vi "Get TableName.vi"(8 "error in (no error)":errorcluster caption="entrée d'erreur (pas d'erreur)", 11 "Database Drivers en entrée":refnum<class "Database Drivers.lvclass">) -> (0 "error out":errorcluster caption="sortie d'erreur", 2 "TableName":string, 3 "Database Drivers en sortie":refnum<class "Database Drivers.lvclass">)   [LabVIEW 2020, in "Library Instrument & Equipement.lvlib" / "Library Database.lvlib" / "Database Drivers.lvclass"]
uses:
  Database Drivers.lvclass
  Database Drivers.lvclass/Database Drivers.ctl
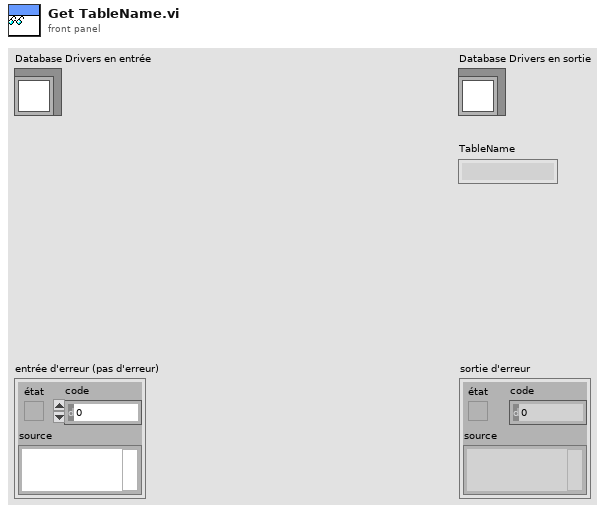
[diagram p1: front panel]
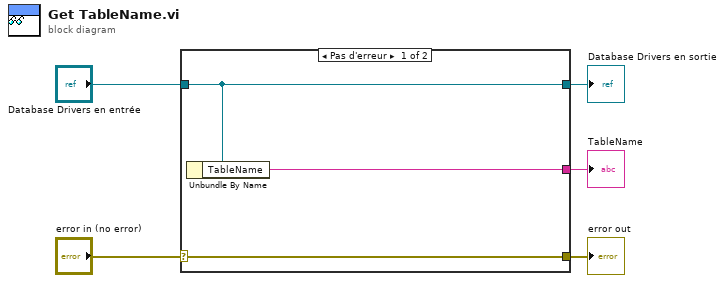
[diagram p0: block diagram]
diagram:
  n1 = case shown="Pas d'erreur" "error in (no error)" {
    selector: "error in (no error)" -> [w8 w9]
    tunnel: [w8 w9] -> w4
    tunnel: [w7 w10] -> w2
    tunnel: "Database Drivers en entrée" -> [w7 w10]
    tunnel: [w6 _] -> w1
    frame No Error {
      n2 = Unbundle By Name(w7) -> ("TableName"=w6:string)
    }
    frame Error {
    }
  }
  "error out" <- w4
  "Database Drivers en sortie" <- w2
  "TableName" <- w1
